vi "z_init.vi"(9 "z comp":dbl[][](array[numeric]), 10 "xy in":dbl[][](array[numeric]), 11 "z in":dbl[](array[numeric])) -> (3 "z":dbl[](array[numeric]))   [LabVIEW 2013]
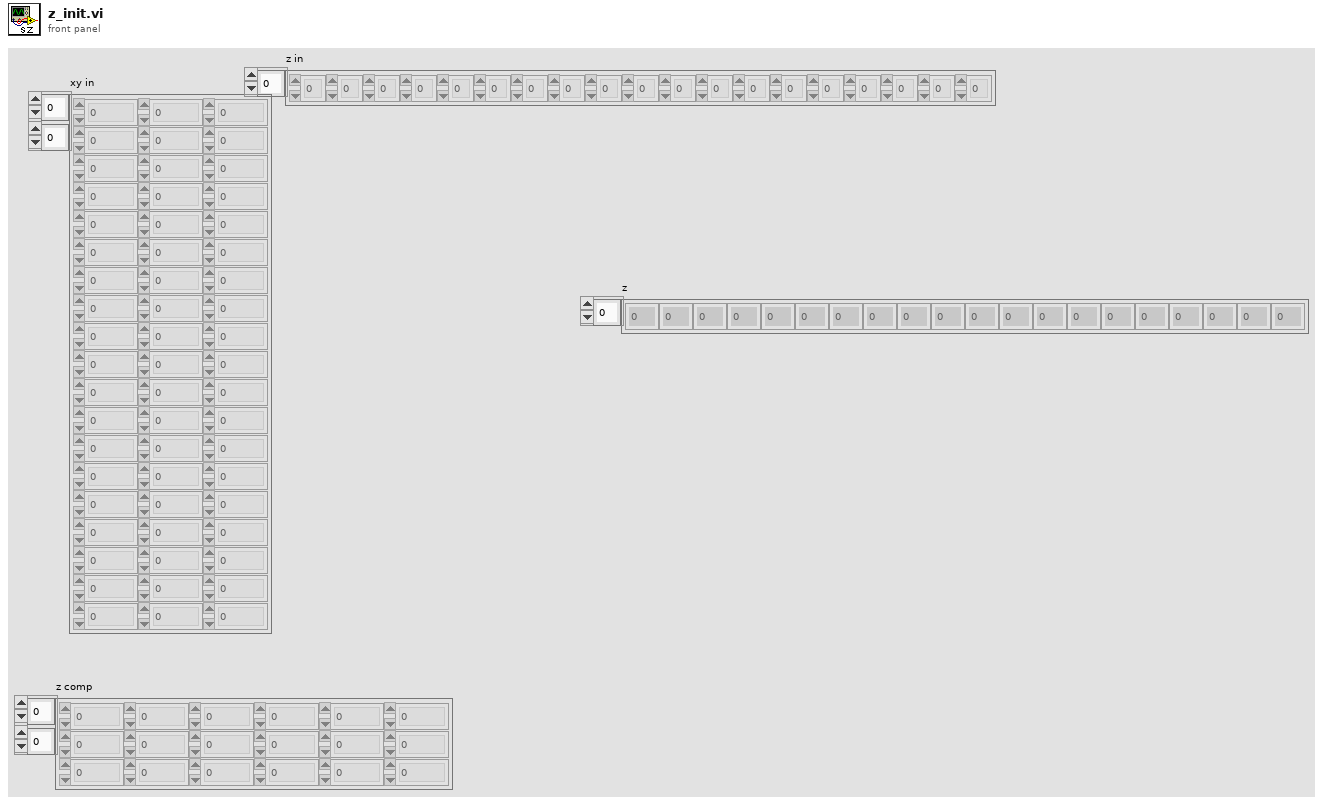
[diagram p1: front panel]
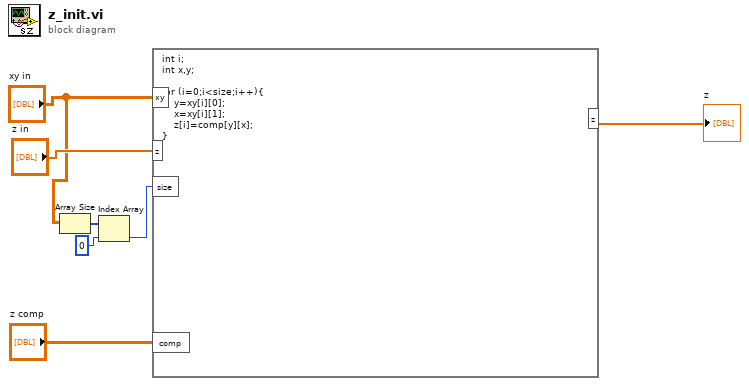
[diagram p0: block diagram]
diagram:
  n1 = Array Size(array="xy in") -> (size(s)=w3:i32[])
  n2 = Index Array(array=w3, index=0) -> (element=w2:i32)
  n3 = formula code="int i;\nint x,y;\n\nfor (i=0;i<size;i++){\n    y=xy[i][0];\n    x=xy[i][1];\n    z[i]=comp[y][x];\n}"("comp"="z comp", "xy"="xy in", "z"="z in", "size"=w2) -> ("z"=→"z":dbl[])
